vi "setNames.vi"(8 "error in (no error)":errorcluster, 10 "Names":string[](array[string]), 11 "NameIterator in":refnum<class "NameIterator.lvclass">) -> (0 "error out":errorcluster, 3 "NameIterator out":refnum<class "NameIterator.lvclass">)   [LabVIEW 2016, in "NameIterator.lvclass"]
uses:
  NameIterator.lvclass
  NameIterator.lvclass/NameIterator.ctl
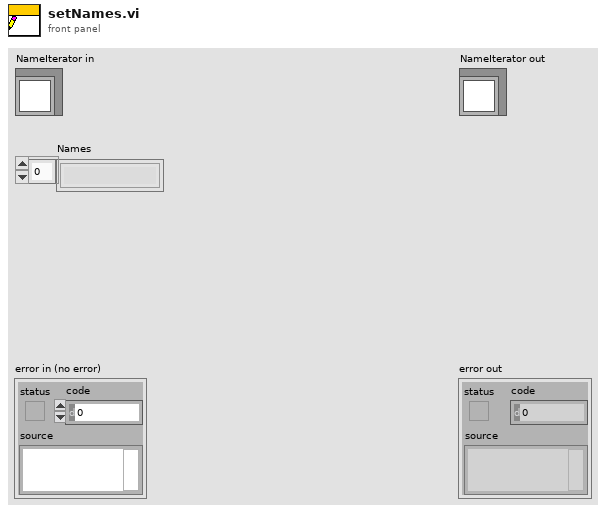
[diagram p1: front panel]
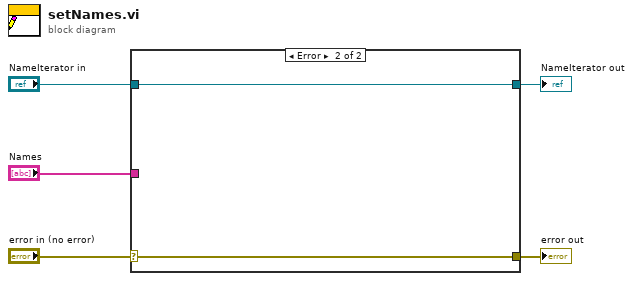
[diagram p0: block diagram]
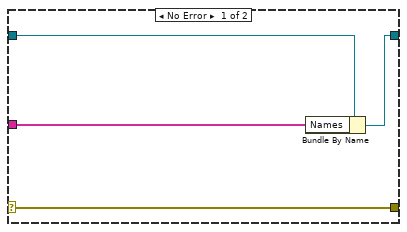
[diagram p2: hidden frame]
diagram:
  n1 = case shown="Error" "error in (no error)" {
    selector: "error in (no error)" -> [w9 w10]
    tunnel: [w9 w10] -> w4
    tunnel: [w7 w11] -> w2
    tunnel: "NameIterator in" -> [w8 w11]
    tunnel: "Names" -> [w6 _]
    frame No Error {
      n2 = Bundle By Name(cluster=w8, "Names"=w6) -> (w7:refnum<class "NameIterator.lvclass">)
    }
    frame Error {
    }
  }
  "error out" <- w4
  "NameIterator out" <- w2
